vi "Main.vi"() -> ()   [LabVIEW 2023, in "Example Plugin.lvclass"]
uses:
  Example Plugin.lvclass
  Example Plugin.lvclass/Example Plugin.ctl
  Capabilities/High Level Capabilities/Device/Device.lvclass
  Capabilities/Low Level Capabilities/Current/Current Actual Value/Current Actual Value.lvclass
panel:
  in  "Actual Value":dbl[](array[numeric])
  out "Voltage.SP":dbl[](array[numeric])
  out "Current.SP":dbl[](array[numeric])
  in  "Example Plugin.lvclass":refnum<class "Example Plugin.lvclass">
  in  "stop":bool
  in  "Number of Channels":u32=1
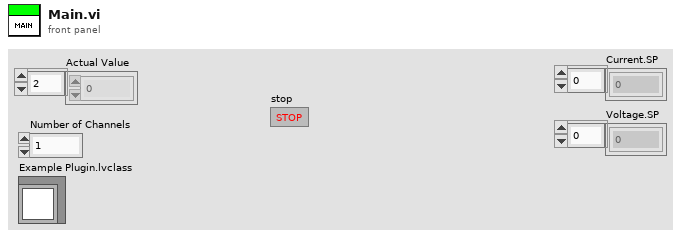
[diagram p1: front panel]
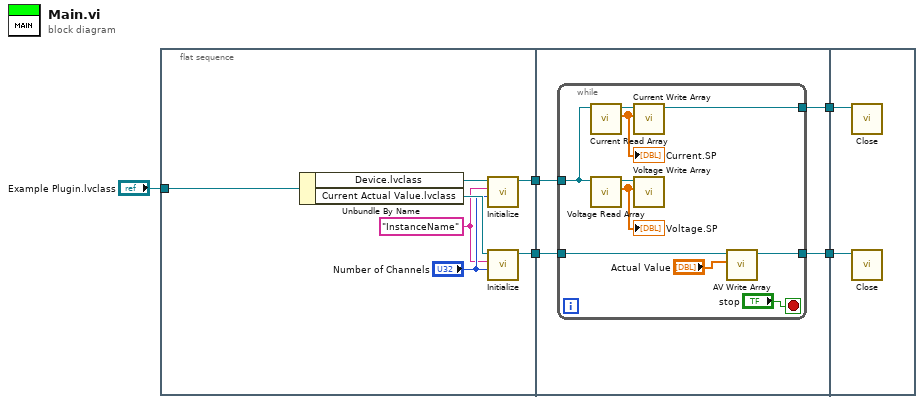
[diagram p0: block diagram]
diagram:
  n1 = flat-sequence {
    tunnel: "Example Plugin.lvclass" -> [w12]
    tunnel: [w11] -> w4
    tunnel: [w6] -> w2
    tunnel: w4 -> [w16]
    tunnel: [w15] -> w3
    tunnel: w2 -> [w14]
    tunnel: [w13] -> w1
    tunnel: w3 -> [w28]
    tunnel: w1 -> [w27]
    frame #0 {
      w7 = "InstanceName" ("Plugin Name")
      n2 = Unbundle By Name(w12) -> ("Device.lvclass"=w10:refnum<class "Device.lvclass">, "Current Actual Value.lvclass"=w9:refnum<class "Current Actual Value.lvclass">)
      n3 = call-dynamic "Initialize.vi"("Number of Channels"="Number of Channels", "Instance Name"=w7, "Device in"=w10) -> ("Device out"=w11:refnum<class "Device.lvclass">)  [unwired: 7 in, 1 out]
      n4 = call-dynamic "Initialize.vi"("Number of Channels"="Number of Channels", "Instance Name"=w7, "Current Actual Value in"=w9) -> ("Current Actual Value out"=w6:refnum<class "Current Actual Value.lvclass">)  [unwired: 7 in, 1 out]
    }
    frame #1 {
      n5 = while {
        tunnel: w16 -> [w22]
        tunnel: [w23] -> w15
        tunnel: w14 -> [w19]
        tunnel: [w17] -> w13
        stop <- "stop" stop-if-true
        n6 = call "Current Read Array.vi"("Device in"=w22) -> ("Current.SP"=w24:dbl[], "Device out"=w25:refnum<class "Device.lvclass">)  [unwired: 9 in]
        "Current.SP" <- w24
        n7 = call "Voltage Read Array.vi"("Device in"=w22) -> ("Voltage.SP"=w20:dbl[], "Device out"=w21:refnum<class "Device.lvclass">)  [unwired: 9 in]
        "Voltage.SP" <- w20
        n8 = call "Current Write Array.vi"("Current.AV"=w24, "Device in"=w25) -> ("Device out"=w23:refnum<class "Device.lvclass">)  [unwired: 9 in]
        n9 = call "Voltage Write Array.vi"("Voltage.AV"=w20, "Device in"=w21) -> ()  [unwired: 9 in, 1 out]
        n10 = call-dynamic "AV Write Array.vi"("Actual Value"="Actual Value", "Actual Value in"=w19) -> ("Actual Value out"=w17:refnum<class "Current Actual Value.lvclass">)  [unwired: 8 in, 1 out]
      }
    }
    frame #2 {
      n11 = call-dynamic "Close.vi"("Device in"=w28) -> ()  [unwired: 9 in, 2 out]
      n12 = call-dynamic "Close.vi"("Actual Value in"=w27) -> ()  [unwired: 9 in, 2 out]
    }
  }
